vi "Process.vi"(8 "error in":errorcluster, 11 "Example Instrument UI":refnum<class "Example Instrument UI.lvclass">) -> (0 "error out":errorcluster, 3 "Example Instrument UI out":refnum<class "Example Instrument UI.lvclass">)   [LabVIEW 2016, in "Example Instrument UI.lvclass"]
doc: "---------------------------------------------------------------\nJKI State Machine Objects™\nhttp://jki.net/state-machine-objects/\nCopyright (C) 2005-2015, JKI <info@jki.net>\nALL RIGHTS RESERVEDJKI State Machine Objects (SMO) 1.0.0.5\nJKI - JKI\nCopyright (c) 2016, JKI"
uses:
  Example Instrument UI.lvclass
  C:/Program Files (x86)/National Instruments/LabVIEW 2016/vi.lib/JKI/JKI SMO/SMO/SMO.lvclass
  C:/Program Files (x86)/National Instruments/LabVIEW 2016/vi.lib/JKI/JKI SMO/SMO.UI/SMO.UI.lvclass
  <vilib>/JKI/JKI SMO/SMO/Typedefs/Parent Call--Enum.ctl
  Example Instrument UI.lvclass/Example Instrument UI.ctl
  Example Instrument/Typedefs/getAll--Cluster.ctl
  <vilib>/JKI/JKI SMO/SMO.UI/SMO.UI.lvclass
  Instrument/Instrument.lvclass
  <vilib>/JKI/JKI SMO/SMO/SMO.lvclass
  Example Instrument/Example Instrument.lvclass
panel:
  out "Numeric":u32
  out "Magnet Return":dbl
  in  "Set Magnet":bool
  in  "Magnet Setpoint":dbl
  in  "STOP":bool
  out "SMO string":string
  out "SMO Boolean":bool
  out "Logger SMO":dbl
  out "Levy 1":dbl
  # "SMO UI Template"
  # "For instructions on how to use the JKI State Machine Objects, examples and video tutorials, visit:\nhttp://jki.net/state-machine-objects/\n\nJKI State Machine Objects™\nhttp://jki.net/state-machine-objects/\nCopyright (C) 2005-2015, JKI <info@jki.net>\nALL RIGHTS RESERVED"
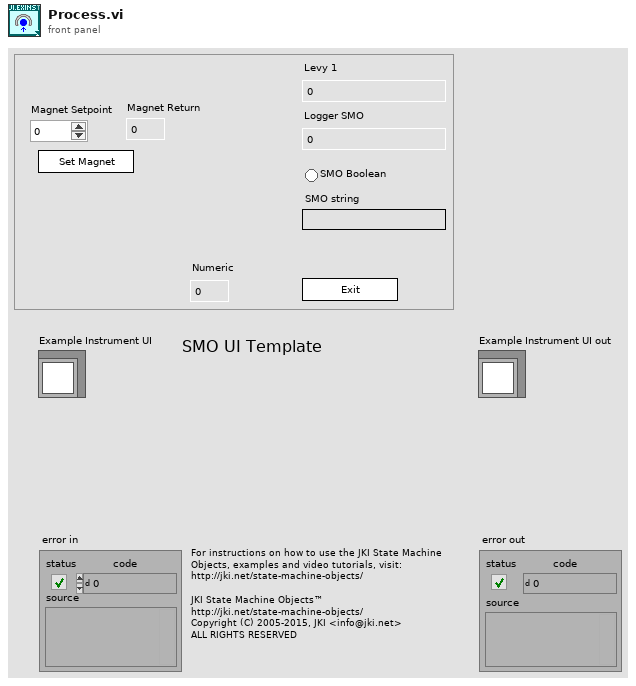
[diagram p1: front panel]
types:
  T1 = typedef "SMO.lvclass/Parent Call--Enum.ctl" = enum16{"Allows parent to run", "Does not request parent to run"}
  T2 = enum32{"invalid app kind", "Development System", "Run Time System", "Student Edition", "Embedded LabVIEW", "Evaluation", "Custom"}
  T3 = enum32{"Invalid", "Standard", "Closed", "Hidden", "Minimized", "Maximized"}
  T4 = typedef "Example Instrument.lvclass/getAll--Cluster.ctl" = cluster{"Levy 1":dbl, "Logger SMO":dbl, "SMO Boolean":bool, "SMO String":string}
  T5 = cluster{"Core":cluster{"Current VI Reference":refnum<vi>, "Close Panel on Exit?":bool, "error":errorcluster}, "Self Reference":refnum<class "Example Instrument UI.lvclass">, "Instrument":refnum<class "Instrument.lvclass">, "getAll":variant, "Magnet Setpoint":dbl}
  T6 = cluster{"Current VI Reference":refnum<vi>, "Close Panel on Exit?":bool, "error":errorcluster}
  T7 = typedef "SMO.lvclass/Protected Events.ctl" = cluster{"StopProcesses":refnum<user-event>, "AbortProcesses":refnum<user-event>, "Config Changed":refnum<user-event>, "Dependency":refnum<user-event>}
  T8 = typedef "Instrument.lvclass/PublicEvents--Cluster.ctl" = cluster{"MessageFromProcess":refnum<user-event>}
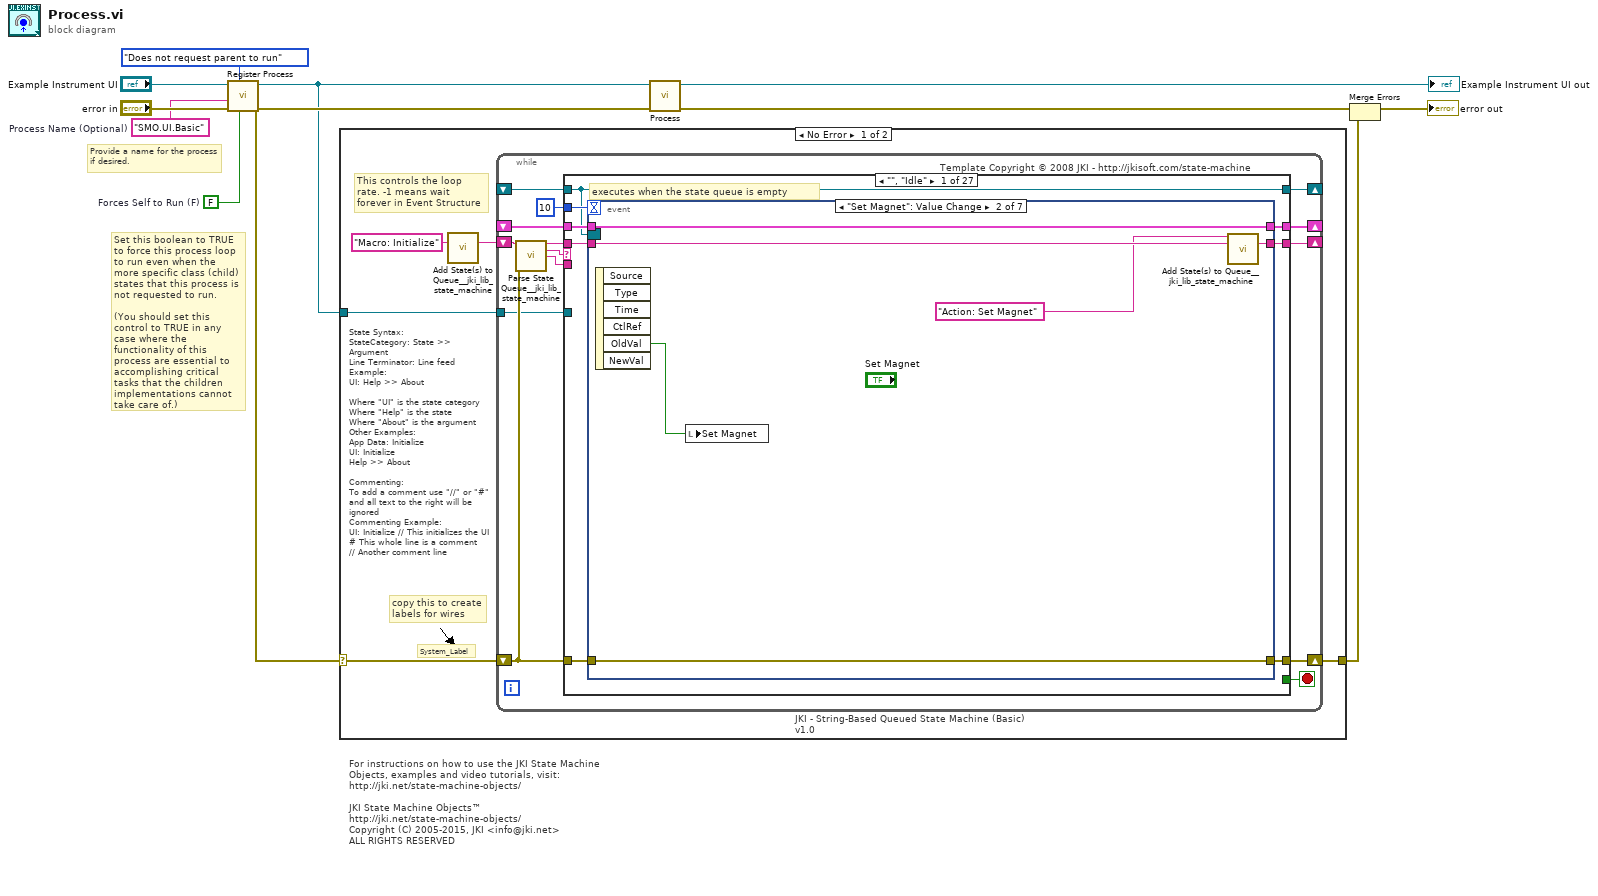
[diagram p0: block diagram]
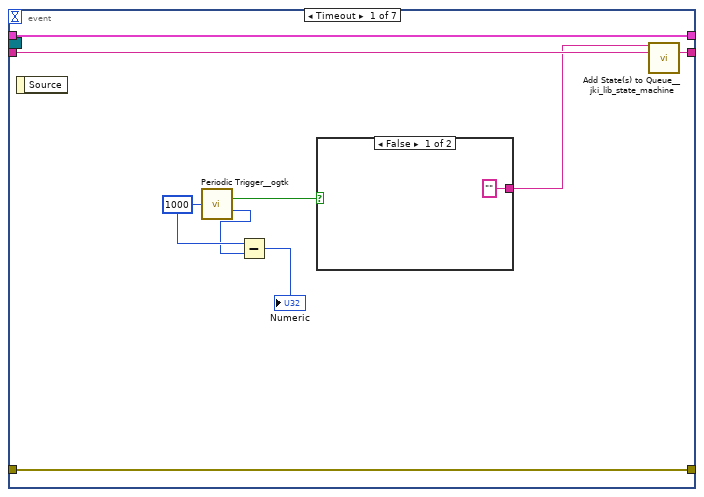
[diagram p2: hidden frame]
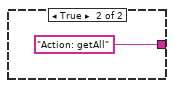
[diagram p3: hidden frame]
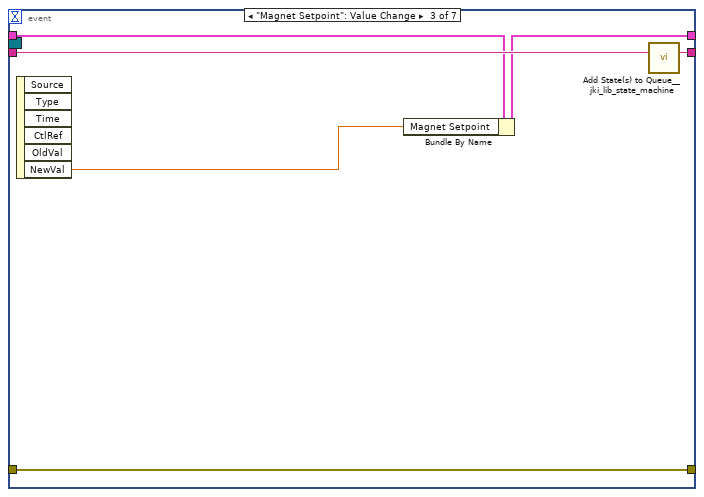
[diagram p4: hidden frame]
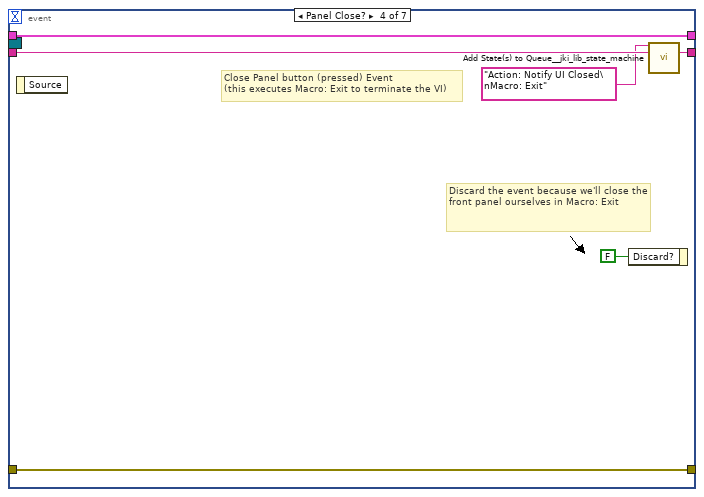
[diagram p5: hidden frame]
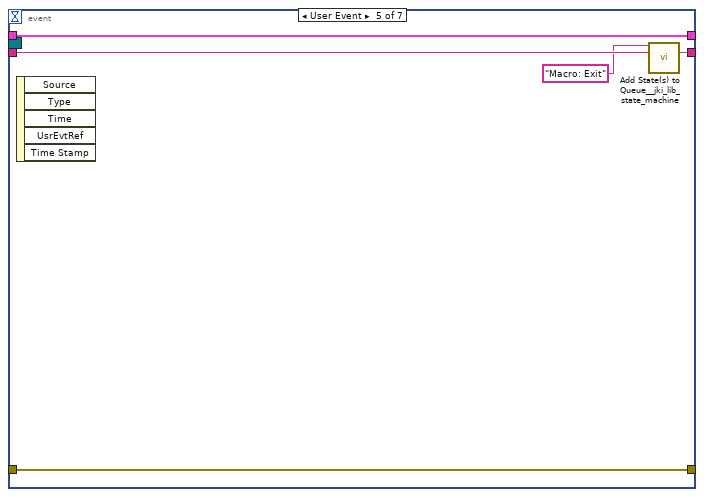
[diagram p6: hidden frame]
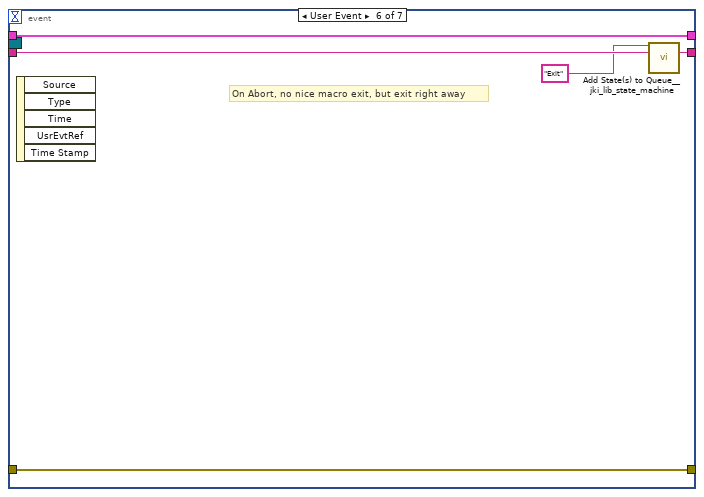
[diagram p7: hidden frame]
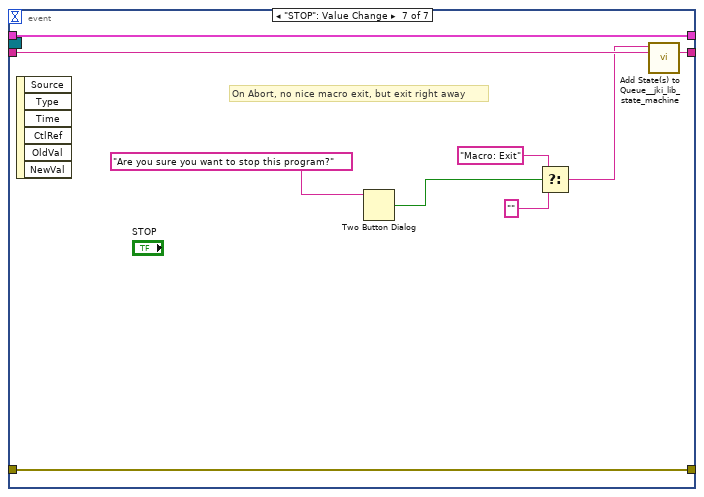
[diagram p8: hidden frame]
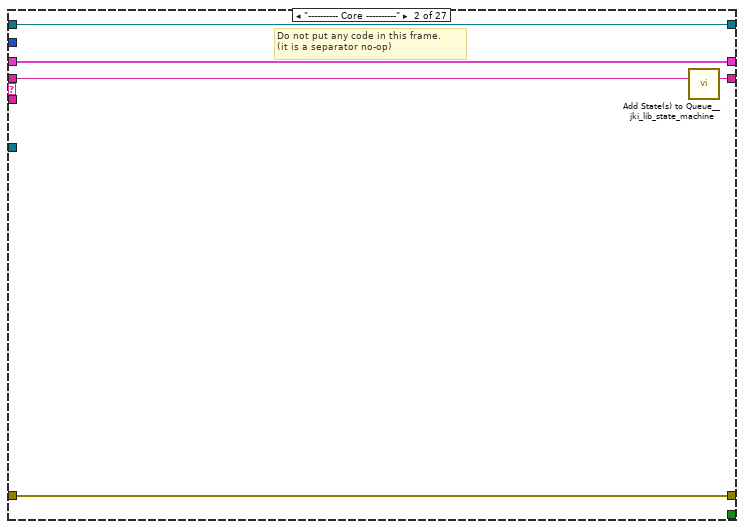
[diagram p9: hidden frame]
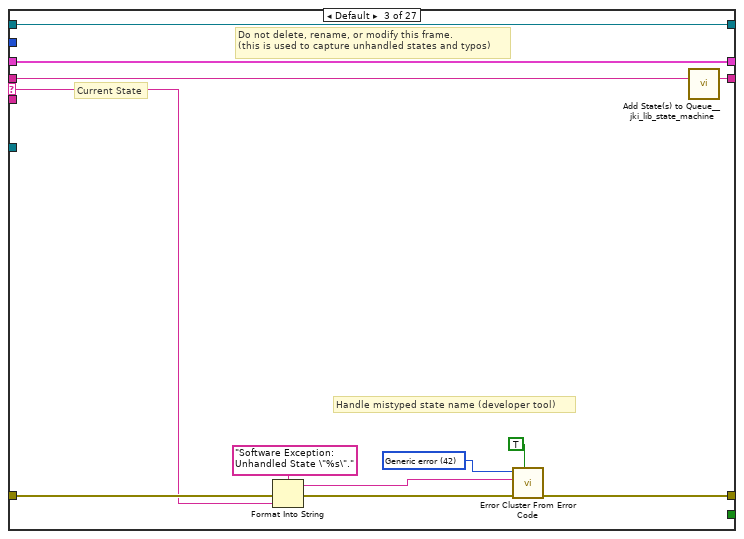
[diagram p10: hidden frame]
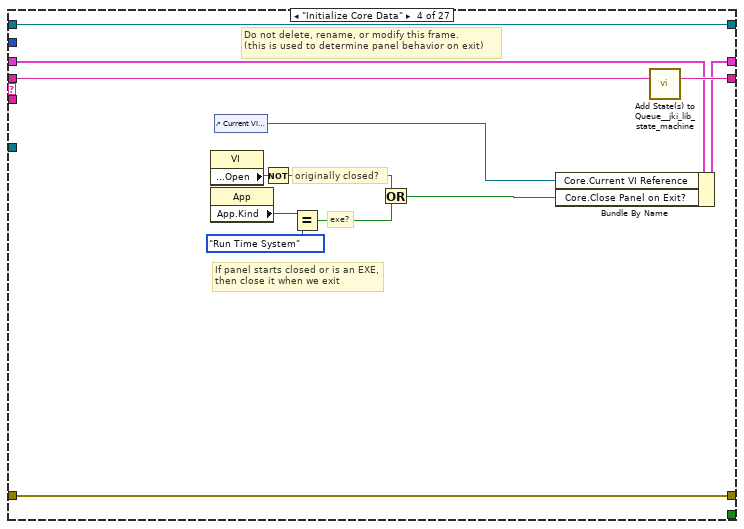
[diagram p11: hidden frame]
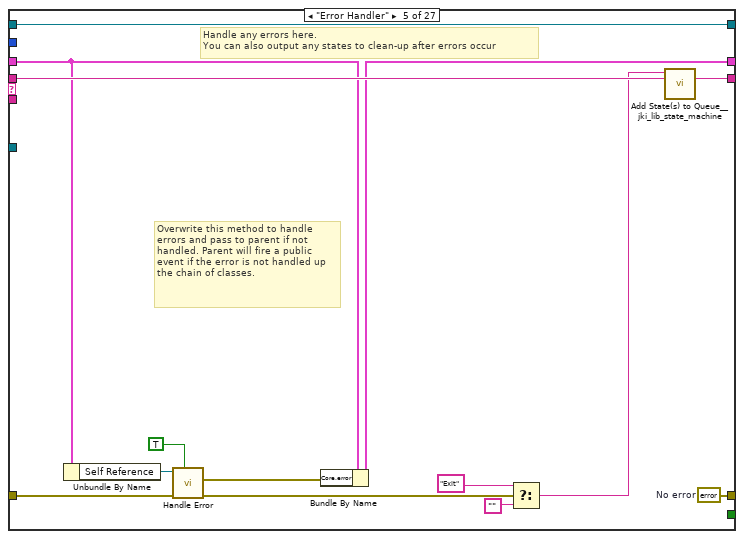
[diagram p12: hidden frame]
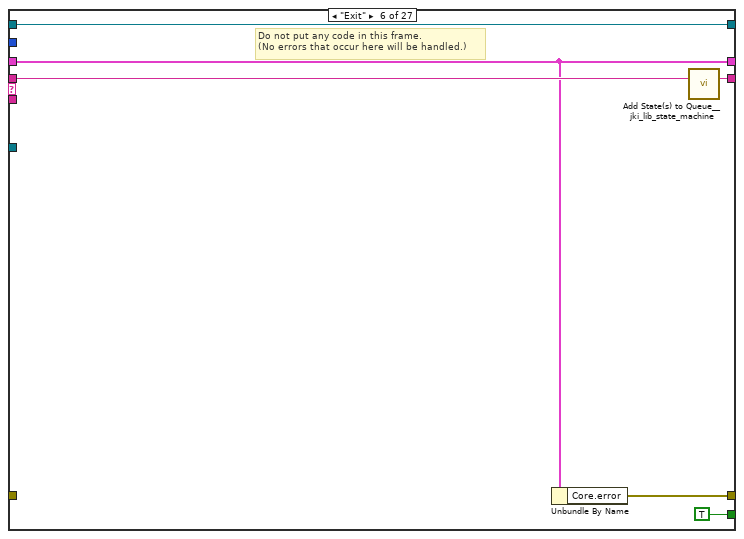
[diagram p13: hidden frame]
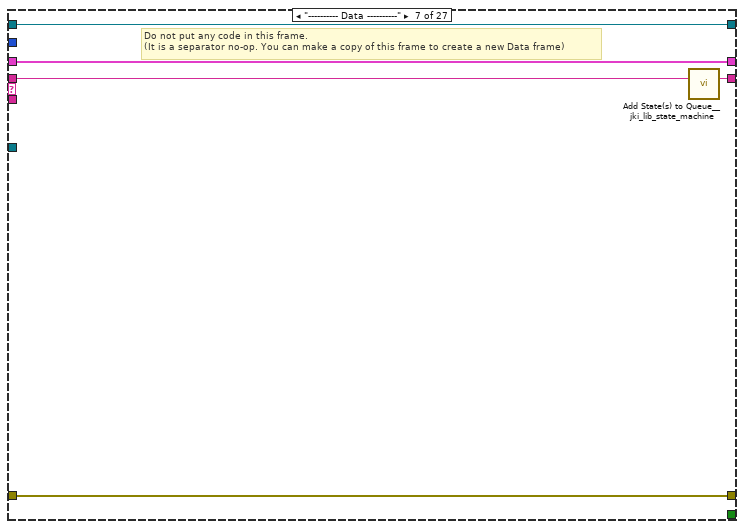
[diagram p14: hidden frame]
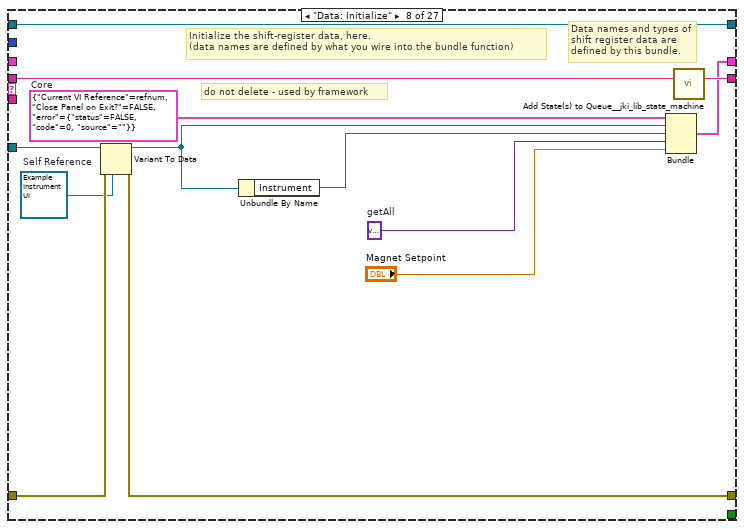
[diagram p15: hidden frame]
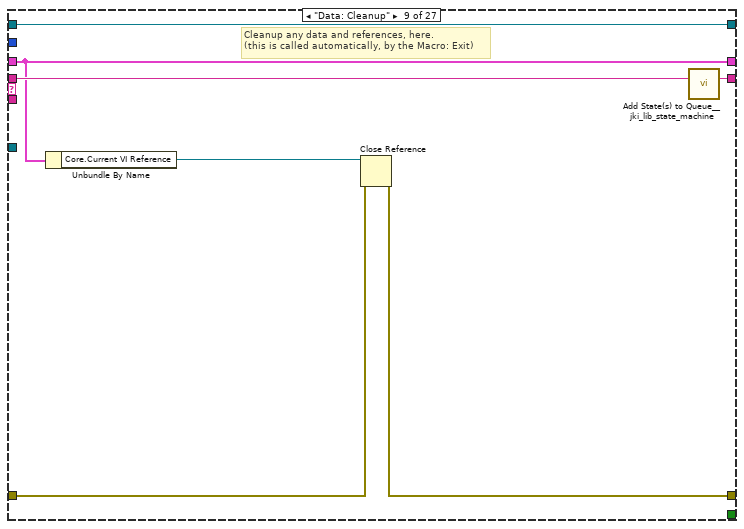
[diagram p16: hidden frame]
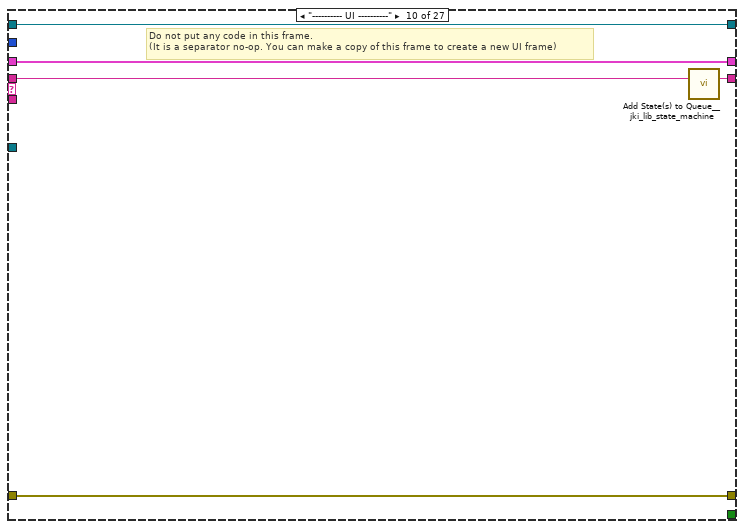
[diagram p17: hidden frame]
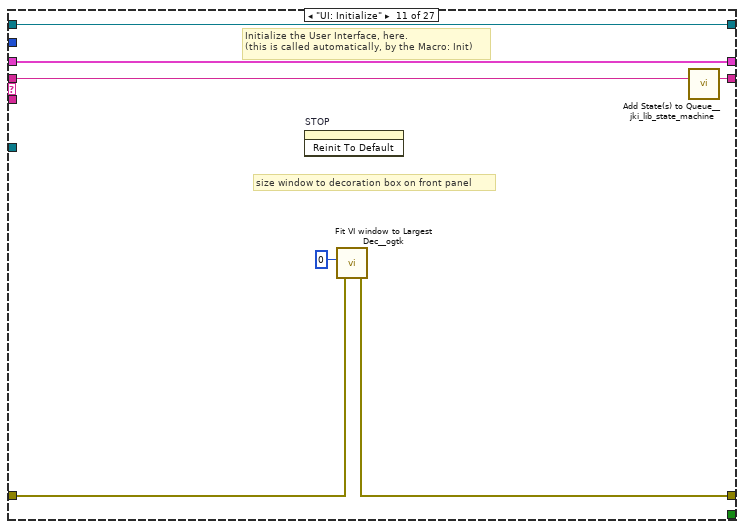
[diagram p18: hidden frame]
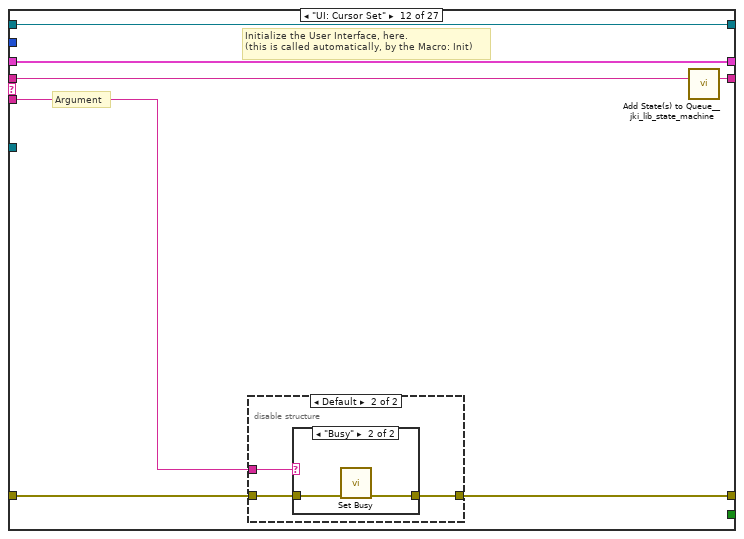
[diagram p19: hidden frame]
diagram:
  w2 = FALSE  # Forces Self to Run (F)
  w1 = "SMO.UI.Basic"  # Process Name (Optional)
  # "Provide a name for the process\nif desired."
  # "Set this boolean to TRUE to force this process loop to run even when the more specific class (child) states that this process is not requested to run.\n\n(You should set this control to TRUE in any case where the functionality of this process are essential to accomplishing critical tasks that the children implementations cannot take care of.)"
  # "For instructions on how to use the JKI State Machine Objects, examples and video tutorials, visit:\nhttp://jki.net/state-machine-objects/\n\nJKI State Machine Objects™\nhttp://jki.net/state-machine-objects/\nCopyright (C) 2005-2015, JKI <info@jki.net>\nALL RIGHTS RESERVED"
  n1 = call <vilib>:"Register Process.vi"("Forces Self to Run (F)"=w2, "Parent Call"=Parent_Call--Enum."Does not request parent to run", "error in (no error)"="error in", "Process Name (optional)"=w1, "SMO"="Example Instrument UI") -> ("error out"=w8:errorcluster, "SMO out"=w7:refnum<class "Example Instrument UI.lvclass">)  [unwired: 5 in]
  n2 = case shown="No Error" w8 {
    selector: w8 -> [w13 w363]
    tunnel: w7 -> [w14 _]
    tunnel: [w12 w363] -> w4
    frame No Error {
      # "State Syntax:\nStateCategory: State >> Argument\nLine Terminator: Line feed\nExample:\nUI: Help >> About\n\nWhere \"UI\" is the state category\nWhere \"Help\" is the state\nWhere \"About\" is the argument\nOther Examples:\nApp Data: Initialize\nUI: Initialize\nHelp >> About\n\nCommenting:\nTo add a comment use \"//\" or \"#\" and all text to the right will be ignored\nCommenting Example:\nUI: Initialize // This initializes the UI\n# This whole line is a comment\n// Another comment line"
      # "copy this to create labels for wires"
      # "This controls the loop rate. -1 means wait forever in Event Structure"
      # "System_Label"
      n3 = call <vilib>:"Add State(s) to Queue__jki_lib_state_machine.vi"("State(s) in (\"\")"="Macro: Initialize") -> ("States Out"=w16:string)  [unwired: 14 in]
      n4 = while "JKI - String-Based Queued State Machine (Basic) v1.0" {
        shift-right: [w23] -> _
        shift-left: _ -> [w22]
        shift-right: [w26] -> w12
        shift-left: w13 -> [w20]
        shift-right: [w25] -> _
        shift-left: w16 -> [w27]
        tunnel: w14 -> [w19]
        shift-right: [w18] -> _
        shift-left: _ -> [w17]
        stop <- w24 stop-if-true
        # "Template Copyright © 2008 JKI - http://jkisoft.com/state-machine"
        n5 = call <vilib>:"Parse State Queue__jki_lib_state_machine.vi"("State Queue"=w27, "Error In (no error)"=w20) -> ("Remaining States"=w29:string, "Current State"=w30:string, "Arguments"=w28:string)  [unwired: 11 in]
        n6 = case shown="\"\", \"Idle\"" w30 {
          selector: w30 -> [_ _ w93 _ _ _ _ _ _ _ _ _ _ _ _ _ _ _ _ _ _ _ _ _ _ _ _]
          tunnel: w29 -> [w38 w91 w97 w116 w130 w136 w141 w154 w161 w166 w173 w180 w196 w228 w237 w251 w256 w267 w274 w279 w292 w298 w305 w312 w325 w339 w356]
          tunnel: w28 -> [_ _ _ _ _ _ _ _ _ _ _ w174 w190 _ _ _ _ _ _ _ _ _ _ _ _ _ _]
          tunnel: w22 -> [w36 w88 w95 w107 w119 w132 w138 _ w156 w163 w171 w178 w192 w225 w233 w242 w253 w264 w269 w276 w290 w296 w301 w308 w322 w336 w353]
          tunnel: [w35 w89 w99 w113 w121 w131 w139 w150 w157 w164 w168 w175 w193 w226 w235 w249 w254 w258 w270 w277 w285 w293 w302 w306 w318 w333 w343] -> w26
          tunnel: w20 -> [w34 w89 w98 w113 w126 _ w139 w151 w158 w164 w169 w176 w194 w226 w235 w249 w254 w259 w271 w277 w287 w294 w302 w307 w319 w333 w344]
          tunnel: [w37 w90 w96 w115 w129 w135 w140 w153 w160 w165 w172 w179 w195 w227 w236 w250 w255 w266 w273 w278 w291 w297 w304 w311 w324 w338 w355] -> w25
          tunnel: [_ _ _ _ _ TRUE _ _ _ _ _ _ _ _ _ _ _ _ _ _ _ _ _ _ _ _ _] -> w24
          tunnel: [w33 w88 w95 w114 w118 w132 w138 w152 w156 w163 w171 w178 w192 w225 w233 w242 w253 w264 w269 w276 w290 w296 w300 w308 w322 w328 w347] -> w23
          tunnel: 10 ("Timeout") -> [w32 _ _ _ _ _ _ _ _ _ _ _ _ _ _ _ _ _ _ _ _ _ _ _ _ _ _]
          tunnel: w19 -> [_ _ _ _ _ _ _ w148 _ _ _ _ _ _ _ _ _ _ _ _ _ _ _ _ _ _ _]
          tunnel: [w31 w87 w92 w104 w128 w133 w137 w147 w155 w162 w170 w177 w189 w224 w234 w243 w252 w265 w272 w275 w289 w295 w303 w310 w323 w337 w354] -> w18
          tunnel: w17 -> [w31 w87 w92 w104 w128 w133 w137 w147 w155 w162 w170 w177 w189 w224 w234 w243 w252 w265 w272 w275 _ w295 w303 w310 w323 w337 w354]
          frame "", "Idle" {
            # "executes when the state queue is empty"
            n7 = event shown="[1] \"Set Magnet\": Value Change" {
              selector: w31 -> [_ _ _ _ _ _ _]
              dyn-events: _ -> [_ _ _ _ _ _ _]
              timeout: w32 -> [_ _ _ _ _ _ _]
              tunnel: w38 -> [w47 w55 w61 w67 w72 w77 w86]
              tunnel: [w46 w54 w60 w66 w71 w76 w85] -> w37
              tunnel: w36 -> [w44 w52 w57 w63 w69 w74 w83]
              tunnel: [w45 w53 w59 w62 w70 w75 w84] -> w35
              tunnel: w34 -> [w45 w53 w59 w62 w70 w75 w84]
              tunnel: [w44 w52 w56 w63 w69 w74 w83] -> w33
              event Timeout {
                w41 = u32 1000 ("time (ms)")
                n8 = event-data() -> ()  [unwired: 1 in, 1 out]
                n9 = call <userlib>:"Periodic Trigger__ogtk.vi"("time (ms)"=w41) -> ("Triggered"=w42:bool, "timer value"=w39:u32)  [unwired: 12 in, 1 out]
                n10 = Subtract(x=w41, y=w39) -> (x-y=→"Numeric":u32)
                n11 = case shown="False" w42 {
                  tunnel: ["" ("State(s) in Front (\"\")") "Action: getAll" ("State(s) in Front (\"\")")] -> w43
                  frame False {
                  }
                  frame True {
                  }
                }
                n12 = call <vilib>:"Add State(s) to Queue__jki_lib_state_machine.vi"("State(s) in Front (\"\")"=w43, "State(s) in (\"\")"=w47) -> ("States Out"=w46:string)  [unwired: 13 in]
              }
              event "Set Magnet": Value Change {
                n13 = event-data() -> ("OldVal"=w50:bool)  [unwired: 1 in, 5 out]
                n14 = local write "Set Magnet"(w50) -> ()
                n15 = call <vilib>:"Add State(s) to Queue__jki_lib_state_machine.vi"("State(s) in Front (\"\")"="Action: Set Magnet" ("State(s) in Front (\"\")"), "State(s) in (\"\")"=w55) -> ("States Out"=w54:string)  [unwired: 13 in]
              }
              event "Magnet Setpoint": Value Change {
                n16 = event-data() -> ("NewVal"=w58:dbl)  [unwired: 1 in, 5 out]
                n17 = Bundle By Name(cluster=w57, "Magnet Setpoint"=w58) -> (w56:T5)
                n18 = call <vilib>:"Add State(s) to Queue__jki_lib_state_machine.vi"("State(s) in (\"\")"=w61) -> ("States Out"=w60:string)  [unwired: 14 in]
              }
              event Panel Close? {
                # "Discard the event because we'll close the front panel ourselves in Macro: Exit"
                # "Close Panel button (pressed) Event\n(this executes Macro: Exit to terminate the VI)"
                n19 = event-data() -> ()  [unwired: 1 in, 1 out]
                n20 = event-data("Discard?"=FALSE) -> ()  [unwired: 1 in, 1 out]
                n21 = call <vilib>:"Add State(s) to Queue__jki_lib_state_machine.vi"("State(s) in Front (\"\")"="Action: Notify UI Closed\nMacro: Exit", "State(s) in (\"\")"=w67) -> ("States Out"=w66:string)  [unwired: 13 in]
              }
              event User Event {
                n22 = event-data() -> ()  [unwired: 1 in, 5 out]
                n23 = call <vilib>:"Add State(s) to Queue__jki_lib_state_machine.vi"("State(s) in Front (\"\")"="Macro: Exit", "State(s) in (\"\")"=w72) -> ("States Out"=w71:string)  [unwired: 13 in]
              }
              event User Event {
                # "On Abort, no nice macro exit, but exit right away"
                n24 = event-data() -> ()  [unwired: 1 in, 5 out]
                n25 = call <vilib>:"Add State(s) to Queue__jki_lib_state_machine.vi"("State(s) in Front (\"\")"="Exit", "State(s) in (\"\")"=w77) -> ("States Out"=w76:string)  [unwired: 13 in]
              }
              event "STOP": Value Change {
                # "On Abort, no nice macro exit, but exit right away"
                n26 = event-data() -> ()  [unwired: 1 in, 6 out]
                n27 = Two Button Dialog(message="Are you sure you want to stop this program?") -> (T button?=w82:bool)  [unwired: 2 in]
                n28 = Select(t="Macro: Exit", s=w82, f="") -> (s? t:f=w78:string)
                n29 = call <vilib>:"Add State(s) to Queue__jki_lib_state_machine.vi"("State(s) in Front (\"\")"=w78, "State(s) in (\"\")"=w86) -> ("States Out"=w85:string)  [unwired: 13 in]
              }
            }
          }
          frame "---------- Core ----------" {
            # "Do not put any code in this frame.\n(it is a separator no-op)"
            n30 = call <vilib>:"Add State(s) to Queue__jki_lib_state_machine.vi"("State(s) in (\"\")"=w91) -> ("States Out"=w90:string)  [unwired: 14 in]
          }
          frame Default {
            w102 = 42 items=["No error", "Argument error", "Memory is full", "Out of zone", "End of file", "File already open", "Generic file I/O error", "File not found", "File permission error", "Disk is full", "Duplicate path", "Too many files open", "System feature not enabled", "Resource file not found", "Cannot add resource", "Resource not found", "Image not found", "Image memory error", "Pen does not exist", "Config type invalid", "Config token not found", "Config parse error", "Config memory error", "Bad external code format", "Bad external code offset", "External code not present", "Null window", "Destroy window error", "Null menu", "Print aborted", "Bad print record", "Print driver error", "Windows error during printing", "Memory error during printing", "Print dialog error", "Generic print error", "Invalid device refnum", "Device not found", "Device parameter error", "Device unit error", "Cannot open device", "Device call aborted", "Generic error", "Cancelled by user", "Object ID too low", "Object ID too high", "Object not in heap", "Unknown heap", "Unknown object (invalid DefProc)", "Unknown object (DefProc not in table)", "Message out of range", "Invalid (null) method", "Unknown message", "Manager call not supported", "Bad address", "Network operation in progress", "Network operation timed out", "Connection is busy", "Network attribute not supported", "Network error", "Address in use", "System out of memory", "Connection aborted", "Connection refused", "Not connected", "Already connected", "Connection closed", "Initialization error (interapplication manager)", "Bad occurrence", "Wait on unbound occurrence handler", "Occurrence queue overflow", "Datalog type conflict", "Unused", "Unrecognized type (interapplication manager)", "Memory corrupt", "Failed to make temporary DLL", "Old CIN version", "Drag socket not found", "Failed to load drop-object", "Failed to register OLE object", "Failed to release OLE object", "Format specifier type mismatch", "Unknown format specifier", "Too few format specifiers", "Too many format specifiers", "Scan failed", "Newer CIN version", "Error converting to variant", "Runtime menu error", "Password tampered", "Variant attribute not found", "Incompatible variant data type", "Event data is not available", "Event Store is not present", "Occurrence is not found", "Event Queue is not created", "Event info is not available", "Refnum passed is NULL", "Error retrieving Class GUID", "Error retrieving CoClass GUID", "Error retrieving TypeLib GUID.", "Bad built application magic bytes.", "Specific driver is different from the specific driver associated with the Logical Name.", "There is no session opened to the class driver.", "Max Error", "MAX - Error with config objects", "MAX - Error loading configuration", "MAX - Group not supported"]
            # "Current State"
            # "Do not delete, rename, or modify this frame.\n(this is used to capture unhandled states and typos)"
            # "Handle mistyped state name (developer tool)"
            n31 = Format Into String(format string="Software Exception: Unhandled State \"%s\"." ("message"), error in=w98, w93) -> (resulting string=w101:string, error out=w100:errorcluster)  [unwired: 1 in]
            n32 = call <vilib>:"Error Cluster From Error Code.vi"("show call chain? (False)"=TRUE, "error in (no error)"=w100, "error message (\"\")"=w101, "error code (0)"=w102) -> ("error out"=w99:errorcluster)  [unwired: 5 in]
            n33 = call <vilib>:"Add State(s) to Queue__jki_lib_state_machine.vi"("State(s) in (\"\")"=w97) -> ("States Out"=w96:string)  [unwired: 14 in]
          }
          frame "Initialize Core Data" {
            # "Do not delete, rename, or modify this frame.\n(this is used to determine panel behavior on exit)"
            # "originally closed?"
            # "exe?"
            # "If panel starts closed or is an EXE, then close it when we exit"
            n34 = property class="VI"() -> ("Front Panel.Open"=w112:bool)  [unwired: 2 in, 2 out]
            n35 = property class="App"() -> ("App.Kind"=w111:T2)  [unwired: 2 in, 2 out]
            n36 = control-ref of="Current VI Reference"() -> (w105:refnum<vi>)
            n37 = Not(x=w112) -> (.not. x?=w109:bool)
            n38 = Equal?(x=w111, y=T2."Run Time System" ("Application:Kind")) -> (x = y?=w108:bool)
            n39 = Or(x=w109, y=w108) -> (x .or. y?=w106:bool)
            n40 = Bundle By Name(cluster=w107, "Core.Current VI Reference"=w105, "Core.Close Panel on Exit?"=w106) -> (w114:T5)
            n41 = call <vilib>:"Add State(s) to Queue__jki_lib_state_machine.vi"("State(s) in (\"\")"=w116) -> ("States Out"=w115:string)  [unwired: 14 in]
          }
          frame "Error Handler" {
            w121 = errorcluster {"status"=FALSE, "code"=0, "source"=""}  # No error
            # "Overwrite this method to handle errors and pass to parent if not handled. Parent will fire a public event if the error is not handled up the chain of classes."
            # "Handle any errors here.\nYou can also output any states to clean-up after errors occur"
            n42 = Unbundle By Name(w119) -> ("Self Reference"=w127:refnum<class "Example Instrument UI.lvclass">)
            n43 = call-dynamic "Handle Error.vi"("Stop on Unhandled Error (T)"=TRUE, "error in"=w126, "SMO"=w127) -> ("handling error"=w122:errorcluster, "Unhandled error"=w120:errorcluster)  [unwired: 6 in, 1 out]
            n44 = Bundle By Name(cluster=w119, "Core.error"=w120) -> (w118:T5)
            n45 = Select(t="Exit", s=w122, f="") -> (s? t:f=w123:string)
            n46 = call <vilib>:"Add State(s) to Queue__jki_lib_state_machine.vi"("State(s) in Front (\"\")"=w123, "State(s) in (\"\")"=w130) -> ("States Out"=w129:string)  [unwired: 13 in]
          }
          frame "Exit" {
            # "Do not put any code in this frame.\n(No errors that occur here will be handled.)"
            n47 = Unbundle By Name(w132) -> ("Core.error"=w131:errorcluster)
            n48 = call <vilib>:"Add State(s) to Queue__jki_lib_state_machine.vi"("State(s) in (\"\")"=w136) -> ("States Out"=w135:string)  [unwired: 14 in]
          }
          frame "---------- Data ----------" {
            # "Do not put any code in this frame.\n(It is a separator no-op. You can make a copy of this frame to create a new Data frame)"
            n49 = call <vilib>:"Add State(s) to Queue__jki_lib_state_machine.vi"("State(s) in (\"\")"=w141) -> ("States Out"=w140:string)  [unwired: 14 in]
          }
          frame "Data: Initialize" {
            w143 = variant  # getAll
            w146 = T6 {"Current VI Reference"=refnum, "Close Panel on Exit?"=FALSE, "error"={"status"=FALSE, "code"=0, "source"=""}}  # Core
            w149 = refnum<class "Example Instrument UI.lvclass"> refnum  # Self Reference
            # "do not delete - used by framework"
            # "Data names and types of shift register data are defined by this bundle."
            # "Initialize the shift-register data, here.\n(data names are defined by what you wire into the bundle function)"
            n50 = Variant To Data(error in=w151, type=w149, Variant=w148) -> (data=w145:refnum<class "Example Instrument UI.lvclass">, error out=w150:errorcluster)
            n51 = Unbundle By Name(w145) -> ("Instrument"=w144:refnum<class "Instrument.lvclass">)
            n52 = Bundle("Core"=w146, "Self Reference"=w145, "Instrument"=w144, "getAll"=w143, "Magnet Setpoint"="Magnet Setpoint") -> (w152:T5)  [unwired: 1 in]
            n53 = call <vilib>:"Add State(s) to Queue__jki_lib_state_machine.vi"("State(s) in (\"\")"=w154) -> ("States Out"=w153:string)  [unwired: 14 in]
          }
          frame "Data: Cleanup" {
            # "Cleanup any data and references, here.\n(this is called automatically, by the Macro: Exit)"
            n54 = Unbundle By Name(w156) -> ("Core.Current VI Reference"=w159:refnum<vi>)
            n55 = Close Reference(reference=w159, error in (no error)=w158) -> (error out=w157:errorcluster)
            n56 = call <vilib>:"Add State(s) to Queue__jki_lib_state_machine.vi"("State(s) in (\"\")"=w161) -> ("States Out"=w160:string)  [unwired: 14 in]
          }
          frame "---------- UI ----------" {
            # "Do not put any code in this frame.\n(It is a separator no-op. You can make a copy of this frame to create a new UI frame)"
            n57 = call <vilib>:"Add State(s) to Queue__jki_lib_state_machine.vi"("State(s) in (\"\")"=w166) -> ("States Out"=w165:string)  [unwired: 14 in]
          }
          frame "UI: Initialize" {
            # "size window to decoration box on front panel"
            # "Initialize the User Interface, here.\n(this is called automatically, by the Macro: Init)"
            n58 = invoke on="STOP" class="Bool (strict)" method="Reinit To Default"() -> ()  [unwired: 3 in, 3 out]
            n59 = call <userlib>:"Fit VI window to Largest Dec__ogtk.vi"("error in (no error)"=w169, "border spacing (2 px)"=0) -> ("error out"=w168:errorcluster)  [unwired: 4 in, 1 out]
            n60 = call <vilib>:"Add State(s) to Queue__jki_lib_state_machine.vi"("State(s) in (\"\")"=w173) -> ("States Out"=w172:string)  [unwired: 14 in]
          }
          frame "UI: Cursor Set" {
            # "Argument"
            # "Initialize the User Interface, here.\n(this is called automatically, by the Macro: Init)"
            n61 = disable-structure shown="Default" {
              disable-tunnel: w176 -> [w181 w184]
              disable-tunnel: [w181 w183] -> w175
              disable-tunnel: w174 -> [_ w182]
              frame condition #0 {
              }
              frame condition #1 (active) {
                n62 = case shown="\"Busy\"" w182 {
                  tunnel: w184 -> [w186 w188]
                  tunnel: [w185 w187] -> w183
                  frame "Idle", Default {
                    n63 = call <vilib>:"Unset Busy.vi"("error in (no error)"=w186) -> ("error out"=w185:errorcluster)  [unwired: 10 in]
                  }
                  frame "Busy" {
                    n64 = call <vilib>:"Set Busy.vi"("error in (no error)"=w188) -> ("error out"=w187:errorcluster)  [unwired: 9 in, 1 out]
                  }
                }
              }
            }
            n65 = call <vilib>:"Add State(s) to Queue__jki_lib_state_machine.vi"("State(s) in (\"\")"=w180) -> ("States Out"=w179:string)  [unwired: 14 in]
          }
          frame "UI: Front Panel State" {
            # "Argument"
            # "Set Front Panel Open or Closed\n(Usage: \"UI: Front Panel State >> Open|Close\")"
            n66 = Unbundle By Name(w192) -> ("Core.Current VI Reference"=w191:refnum<vi>)
            n67 = disable-structure shown="Default" {
              disable-tunnel: w194 -> [w200 w223]
              disable-tunnel: [w199 w223] -> w193
              disable-tunnel: w191 -> [w198 _]
              disable-tunnel: w190 -> [w197 _]
              frame condition #0 (active) {
                n68 = case shown="\"Close\"" w197 {
                  tunnel: w200 -> [w204 w217]
                  tunnel: [w206 w218] -> w199
                  tunnel: w198 -> [w205 w215]
                  frame "Open", Default {
                    n69 = property class="VI"(reference=w205, error in=w204) -> (reference out=w202:refnum<vi>, error out=w203:errorcluster, "FP.State"=w201:T3)
                    n70 = case shown="\"Closed\"" w201 {
                      tunnel: [w209 w212] -> w206
                      tunnel: w203 -> [w208 w212]
                      tunnel: w202 -> [w207 _]
                      frame "Closed" {
                        n71 = invoke class="VI" method="FP.Open"(reference=w207, error in=w208, "Activate"=TRUE, "State"=T3."Standard") -> (error out=w209:errorcluster)  [unwired: 1 in, 4 out]
                      }
                      frame Default {
                      }
                    }
                  }
                  frame "Close" {
                    n72 = property class="VI"(reference=w215, error in=w217) -> (reference out=w214:refnum<vi>, error out=w216:errorcluster, "FP.State"=w213:T3)
                    n73 = case shown="Default" w213 {
                      tunnel: [w219 w222] -> w218
                      tunnel: w216 -> [w219 w221]
                      tunnel: w214 -> [_ w220]
                      frame "Invalid", "Closed" {
                      }
                      frame Default {
                        n74 = invoke class="VI" method="FP.Close"(reference=w220, error in=w221) -> (error out=w222:errorcluster)  [unwired: 1 in, 2 out]
                      }
                    }
                  }
                }
              }
              frame condition #1 {
              }
            }
            n75 = call <vilib>:"Add State(s) to Queue__jki_lib_state_machine.vi"("State(s) in (\"\")"=w196) -> ("States Out"=w195:string)  [unwired: 14 in]
          }
          frame "---------- Macro ----------" {
            # "Do not put any code in this frame.\n(It is a separator no-op. You can make a copy of this frame to create a new Macro frame)"
            n76 = call <vilib>:"Add State(s) to Queue__jki_lib_state_machine.vi"("State(s) in (\"\")"=w228) -> ("States Out"=w227:string)  [unwired: 14 in]
          }
          frame "Macro: Initialize" {
            w231 = "UI: Initialize\n//UI: Front Panel State >> Open"  # UI: Initialize //UI: Front Panel State >> Open
            # "Initialization Macro\n(This is called once, when the VI starts)"
            n77 = call <vilib>:"Add State(s) to Queue__jki_lib_state_machine.vi"("State(s) in Front (\"\")"="Data: Initialize\nInitialize Core Data\nEvents: Register", "State(s) in (\"\")"="Process: Sync", "State(s) at Back (\"\")"=w231) -> ("States Out"=w230:string)  [unwired: 12 in]
            n78 = call <vilib>:"Add State(s) to Queue__jki_lib_state_machine.vi"("State(s) in Front (\"\")"=w230, "State(s) in (\"\")"=w237) -> ("States Out"=w236:string)  [unwired: 13 in]
          }
          frame "Macro: Exit" {
            # "Exit Macro\n(This is called once, when the VI exits)"
            n79 = Unbundle By Name(w242) -> ("Core.Close Panel on Exit?"=w248:bool)
            n80 = Select(t="//UI: Front Panel State >> Close", s=w248, f="") -> (s? t:f=w245:string)
            n81 = call <vilib>:"Add State(s) to Queue__jki_lib_state_machine.vi"("State(s) in Front (\"\")"="Data: Cleanup\nEvents: Unregister\nProcess: Self Terminate", "State(s) in (\"\")"="Process: Sync", "State(s) at Back (\"\")"="Exit") -> ("States Out"=w239:string)  [unwired: 12 in]
            n82 = call <vilib>:"Add State(s) to Queue__jki_lib_state_machine.vi"("State(s) in (\"\")"=w245, "State(s) at Back (\"\")"=w239) -> ("States Out"=w244:string)  [unwired: 13 in]
            n83 = call <vilib>:"Add State(s) to Queue__jki_lib_state_machine.vi"("State(s) in Front (\"\")"=w244, "State(s) in (\"\")"=w251) -> ("States Out"=w250:string)  [unwired: 13 in]
          }
          frame "---------- Process ----------" {
            # "Template Separator\n(You can make a copy of, or modify, this frame)"
            n84 = call <vilib>:"Add State(s) to Queue__jki_lib_state_machine.vi"("State(s) in (\"\")"=w256) -> ("States Out"=w255:string)  [unwired: 14 in]
          }
          frame "Process: Sync" {
            n85 = Unbundle By Name(w264) -> ("Self Reference"=w260:refnum<class "Example Instrument UI.lvclass">)
            n86 = call <vilib>:"WaitOnProcessSync.vi"("error in (no error)"=w259, "SMO"=w260) -> ("error out"=w258:errorcluster, "Don't run?"=w263:bool)  [unwired: 7 in, 1 out]
            n87 = Select(t="Data: Cleanup\nEvents: Unregister\nExit", s=w263, f="") -> (s? t:f=w257:string)
            n88 = call <vilib>:"Add State(s) to Queue__jki_lib_state_machine.vi"("State(s) in Front (\"\")"=w257, "State(s) in (\"\")"=w267) -> ("States Out"=w266:string)  [unwired: 13 in]
          }
          frame "Process: Self Terminate" {
            n89 = Unbundle By Name(w269) -> ("Self Reference"=w268:refnum<class "Example Instrument UI.lvclass">)
            n90 = call <vilib>:"SelfTerminate.vi"("error in (no error)"=w271, "SMO in"=w268) -> ("error out"=w270:errorcluster)  [unwired: 8 in, 1 out]
            n91 = call <vilib>:"Add State(s) to Queue__jki_lib_state_machine.vi"("State(s) in (\"\")"=w274) -> ("States Out"=w273:string)  [unwired: 14 in]
          }
          frame "---------- Events ----------" {
            # "Template Separator\n(You can make a copy of, or modify, this frame)"
            n92 = call <vilib>:"Add State(s) to Queue__jki_lib_state_machine.vi"("State(s) in (\"\")"=w279) -> ("States Out"=w278:string)  [unwired: 14 in]
          }
          frame "Events: Register" {
            # "Expand to add\nmore events"
            # "Base Class Protected Events"
            n93 = Unbundle By Name(w290) -> ("Self Reference"=w283:refnum<class "Example Instrument UI.lvclass">, "Instrument"=w282:refnum<class "Instrument.lvclass">)
            n94 = call <vilib>:"GetProtectedEvents.vi"("SMO"=w283) -> ("error out"=w284:errorcluster, "SMO Protected Events"=w288:T7)  [unwired: 8 in, 1 out]
            n95 = call "Instrument.GetPublicEvents.vi"("Instrument"=w282) -> ("error out"=w280:errorcluster, "Instrument Public Events"=w281:T8)  [unwired: 8 in, 1 out]
            n96 = register-events(w288, w281) -> (reference out=w289:refnum<event-registration>, error out=w286:errorcluster)  [unwired: 2 in]
            n97 = Merge Errors(w280, w287, w286, w284) -> (w285:errorcluster)
            n98 = call <vilib>:"Add State(s) to Queue__jki_lib_state_machine.vi"("State(s) in (\"\")"=w292) -> ("States Out"=w291:string)  [unwired: 14 in]
          }
          frame "Events: Unregister" {
            n99 = Unregister For Events(event registration refnum=w295, error in=w294) -> (error out=w293:errorcluster)
            n100 = call <vilib>:"Add State(s) to Queue__jki_lib_state_machine.vi"("State(s) in (\"\")"=w298) -> ("States Out"=w297:string)  [unwired: 14 in]
          }
          frame "---------- Action ----------" {
            n101 = Unbundle By Name(w301) -> ("Self Reference"=w299:refnum<class "Example Instrument UI.lvclass">)
            n102 = Bundle By Name(cluster=w301, "Self Reference"=w299) -> (w300:T5)
            n103 = call <vilib>:"Add State(s) to Queue__jki_lib_state_machine.vi"("State(s) in (\"\")"=w305) -> ("States Out"=w304:string)  [unwired: 14 in]
          }
          frame "Action: Notify UI Closed" {
            # "Notify that the UI has been closed"
            n104 = Unbundle By Name(w308) -> ("Self Reference"=w309:refnum<class "Example Instrument UI.lvclass">)
            n105 = call <vilib>:"Hide.vi"("error in (no error)"=w307, "SMO.UI"=w309) -> ("error out"=w306:errorcluster)  [unwired: 8 in, 1 out]
            n106 = call <vilib>:"Add State(s) to Queue__jki_lib_state_machine.vi"("State(s) in (\"\")"=w312) -> ("States Out"=w311:string)  [unwired: 14 in]
          }
          frame "Action: Update Front Panel" {
            # "do this way to have nicer UI or only display what you want"
            # "typedef from Child Instrument"
            n107 = Unbundle By Name(w322) -> ("getAll"=w321:variant)
            n108 = Variant To Data(error in=w319, type=T4 {"Levy 1"=0.0, "Logger SMO"=0.0, "SMO Boolean"=FALSE, "SMO String"=""} ("getAll"), Variant=w321) -> (data=w317:T4, error out=w318:errorcluster)
            n109 = Unbundle By Name(w317) -> ("Levy 1"=→"Levy 1":dbl, "Logger SMO"=→"Logger SMO":dbl, "SMO Boolean"=→"SMO Boolean":bool, "SMO String"=→"SMO string":string)
            n110 = call <vilib>:"Add State(s) to Queue__jki_lib_state_machine.vi"("State(s) in (\"\")"=w325) -> ("States Out"=w324:string)  [unwired: 14 in]
          }
          frame "Action: getAll" {
            n111 = Unbundle By Name(w336) -> ("Self Reference"=w335:refnum<class "Example Instrument UI.lvclass">, "Instrument"=w334:refnum<class "Instrument.lvclass">)  [unwired: 1 out]
            n112 = call-dynamic "Remote Client.vi"("Wait for Response?"=TRUE, "error in (no error)"=w333, "Command"="getAll", "Instrument in"=w334) -> ("Data out"=w330:variant, "Command out"=w332:string)  [unwired: 4 in, 2 out]
            n113 = case shown="Default" w332 {
              tunnel: [_ w341] -> w331
              tunnel: w330 -> [_ w341]
              tunnel: [_ "Action: Update Front Panel" ("State(s) in Front (\"\")")] -> w327
              frame Default {
              }
              frame "getAll" {
              }
            }
            n114 = Bundle By Name(cluster=w336, "Self Reference"=w335, "getAll"=w331) -> (w328:T5)
            n115 = call <vilib>:"Add State(s) to Queue__jki_lib_state_machine.vi"("State(s) in Front (\"\")"=w327, "State(s) in (\"\")"=w339) -> ("States Out"=w338:string)  [unwired: 13 in]
          }
          frame "Action: Set Magnet" {
            n116 = Unbundle By Name(w353) -> ("Self Reference"=w352:refnum<class "Example Instrument UI.lvclass">, "Instrument"=w351:refnum<class "Instrument.lvclass">, "Magnet Setpoint"=w346:dbl)
            n117 = call-dynamic "Remote Client.vi"("Wait for Response?"=TRUE, "error in (no error)"=w344, "Data"=w346, "Command"="setMagnet", "Instrument in"=w351) -> ("error out"=w345:errorcluster, "Data out"=w349:variant, "Command out"=w350:string)  [unwired: 3 in, 1 out]
            n118 = case shown="\"setMagnet\"" w350 {
              tunnel: w349 -> [_ w362]
              tunnel: w345 -> [w357 w360]
              tunnel: [w357 w358] -> w343
              frame Default {
              }
              frame "setMagnet" {
                n119 = Variant To Data(error in=w360, type=0.0 ("Magnet Return"), Variant=w362) -> (data=→"Magnet Return":dbl, error out=w358:errorcluster)
              }
            }
            n120 = Bundle By Name(cluster=w353, "Self Reference"=w352) -> (w347:T5)
            n121 = call <vilib>:"Add State(s) to Queue__jki_lib_state_machine.vi"("State(s) in (\"\")"=w356) -> ("States Out"=w355:string)  [unwired: 14 in]
          }
        }
      }
    }
    frame Error {
    }
  }
  n122 = call-parent "Process.vi"("error in (no error)"=w8, "SMO.UI"=w7) -> ("error out"=w5:errorcluster, "SMO.UI out"=→"Example Instrument UI out":refnum<class "Example Instrument UI.lvclass">)  [unwired: 8 in]
  n123 = Merge Errors(w5, w4) -> (→"error out":errorcluster)
